vi "Periodic Tasks.vi"(8 "error in":errorcluster) -> ()   [LabVIEW 2023]
doc: "This VI runs in parallel to other tasks. It can contain as many user-defined periodic loops as you need. These can carry out PID or other sorts of timed response."
uses:
  <vilib>/Rock Robotics/WPI/Utilities/WPI_GetSetVariantRefNum.vi
panel:
  out "Numeric 6":dbl
  out "Numeric 5":dbl
  out "Numeric 4":dbl
  out "Numeric 3":dbl
  out "Numeric 2":dbl
  out "Numeric":dbl
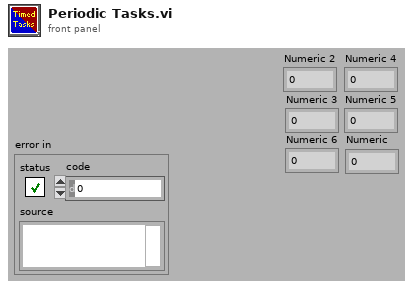
[diagram p1: front panel]
types:
  T1 = typedef "WPI_RobotDriveDevRef.ctl" = cluster{"DevStatus":errorcluster, "Motors[]":T2[], "Square Inputs":bool, "Max Output":dbl}
  T2 = typedef "WPI_MotorControlDeviceRef.ctl" = cluster{"DeviceStatus":errorcluster, "Type":T3, "PWM":cluster{"PWM Channel":T4, "DeadBand":T5}, "CAN":cluster{"Device Number":u8, "SetOutput VI Ref":variant, "GetOutput VI Ref":variant, "Enable VI Ref":variant, "Disable VI Ref":variant, "Data":variant}, "Invert":bool, "DIO PWM":cluster{"PWM \"Enable\" Channel":T4, "DIOChannel":T6, "PWM Rate":dbl}}
  T3 = typedef "WPI_MotorControlType.ctl" = enum16{"PWM", "CAN", "DIO PWM"}
  T4 = typedef "FPGA_DIOPWMChannel.ctl" = enum8{"PWM 0", "PWM 1", "PWM 2", "PWM 3", "PWM 4", "PWM 5", "PWM 6", "PWM 7", "PWM 8", "PWM 9", "PWM MXP 0", "PWM MXP 1", "PWM MXP 2", "PWM MXP 3", "PWM MXP 4", "PWM MXP 5", "PWM MXP 6", "PWM MXP 7", "PWM MXP 8", "PWM MXP 9", "Invalid"}
  T5 = typedef "WPI_PWMDeadband.ctl" = cluster{"Name":string, "maxPositivePwm":i32, "minPositivePwm":i32, "centerPwm":i32, "maxNegativePwm":i32, "minNegativePwm":i32, "angularRange":u16}
  T6 = typedef "FPGA_DIOChannel.ctl" = enum8{"DIO 0", "DIO 1", "DIO 2", "DIO 3", "DIO 4", "DIO 5", "DIO 6", "DIO 7", "DIO 8", "DIO 9", "DIO MXP 0", "DIO MXP 1", "DIO MXP 2", "DIO MXP 3", "DIO MXP 4", "DIO MXP 5", "DIO MXP 6", "DIO MXP 7", "DIO MXP 8", "DIO MXP 9", "DIO MXP 10", "DIO MXP 11", "DIO MXP 12", "DIO MXP 13", "DIO MXP 14", "DIO MXP 15", "SPI Port CS1", "SPI Port CS2", "SPI Port CS3", "SPI Port MISO", "SPI Port MOSI", "Invalid"}
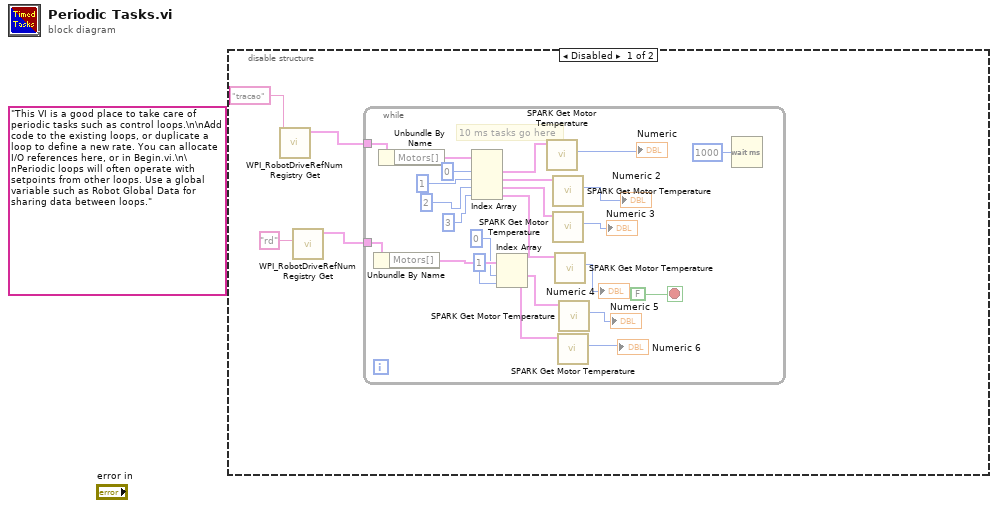
[diagram p0: block diagram]
diagram:
  (unwired) "This VI is a good place to take care of periodic tasks such as control loops.\n\nAdd code to the existing loops, or duplicate a loop to define a new rate. You can allocate I/O references here, or in Begin.vi.\n\nPeriodic loops will often operate with setpoints from other loops. Use a global variable such as Robot Global Data for sharing data between loops."
  n1 = disable-structure shown="Disabled" {
    frame Disabled {
      n2 = call <vilib>:"WPI_RobotDriveRefNum Registry Get.vi"("refnum name"="tracao") -> ("RobotDriveDevRef"=w3:T1)  [unwired: 9 in, 1 out]
      n3 = call <vilib>:"WPI_RobotDriveRefNum Registry Get.vi"("refnum name"="rd") -> ("RobotDriveDevRef"=w1:T1)  [unwired: 9 in, 1 out]
      n4 = while {
        tunnel: w3 -> [w26]
        tunnel: w1 -> [w24]
        stop <- FALSE stop-if-true
        # "10 ms tasks go here"
        n5 = Unbundle By Name(w24) -> ("Motors[]"=w23:T2[])
        n6 = Unbundle By Name(w26) -> ("Motors[]"=w25:T2[])
        n7 = Index Array(array=w25, index #1=0 ("index"), index #2=1 ("index"), index #3=2 ("index"), index #4=3 ("index")) -> (element #1=w16:T2, element #2=w15:T2, element #3=w14:T2, element #4=w13:T2)
        n8 = Index Array(array=w23, index #1=0 ("index"), index #2=1 ("index")) -> (element #1=w8:T2, element #2=w7:T2)
        n9 = call <vilib>:"SPARK Get Motor Temperature.vi"("MotorControlDevRef in"=w16) -> ("Motor Temperature"=→"Numeric":u8)  [unwired: 7 in, 3 out]
        n10 = call <vilib>:"SPARK Get Motor Temperature.vi"("MotorControlDevRef in"=w15) -> ("Motor Temperature"=→"Numeric 2":u8)  [unwired: 7 in, 3 out]
        n11 = call <vilib>:"SPARK Get Motor Temperature.vi"("MotorControlDevRef in"=w14) -> ("Motor Temperature"=→"Numeric 3":u8)  [unwired: 7 in, 3 out]
        n12 = call <vilib>:"SPARK Get Motor Temperature.vi"("MotorControlDevRef in"=w13) -> ("Motor Temperature"=→"Numeric 4":u8)  [unwired: 7 in, 3 out]
        n13 = call <vilib>:"SPARK Get Motor Temperature.vi"("MotorControlDevRef in"=w7) -> ("Motor Temperature"=→"Numeric 6":u8)  [unwired: 7 in, 3 out]
        n14 = call <vilib>:"SPARK Get Motor Temperature.vi"("MotorControlDevRef in"=w8) -> ("Motor Temperature"=→"Numeric 5":u8)  [unwired: 7 in, 3 out]
        n15 = Wait (ms)(milliseconds to wait=u32 1000) -> ()  [unwired: 1 out]
      }
    }
    frame Enabled {
    }
  }
